vi "Preview Test Node.vi"(8 "error in (no error)":errorcluster, 11 "Test Node Model in":refnum<class "Test Node Model.lvclass">) -> (0 "error out":errorcluster, 3 "Test Node Model out":refnum<class "Test Node Model.lvclass">)   [LabVIEW 2013, in "Test Node Model.lvlib" / "Test Node Model.lvclass"]
uses:
  Test Node Model.lvclass
  Test Node Model.lvclass/Test Node Model.ctl
  <vilib>/xml/Load XML File.vi
  <vilib>/xml/Close Reference(Node).vi
  <vilib>/xml/NI_XML.lvlib
  Common/File IO/File IO.lvlib
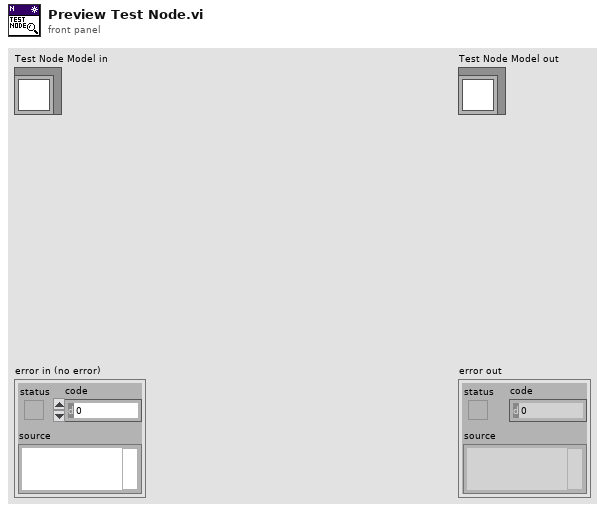
[diagram p1: front panel]
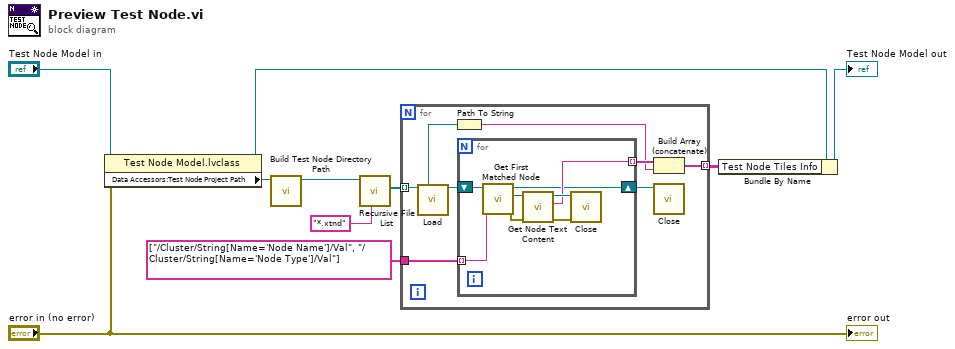
[diagram p0: block diagram]
diagram:
  n1 = property class="Test Node Model.lvclass"(reference="Test Node Model in", error in="error in (no error)") -> (reference out=w8:refnum<class "Test Node Model.lvclass">, "Data Accessors:Test Node Project Path"=w5:path)  [unwired: 1 out]
  n2 = call "Build Test Node Directory Path.vi"("Project Path"=w5) -> ("Test Node Directory Path"=w1:path)  [unwired: 10 in]
  n3 = call <vilib>:"Recursive File List.vi"("pattern"="*.xtnd", "Folder Path"=w1) -> ("All Files in Dir"=w2:path[])  [unwired: 5 in, 4 out]
  n4 = for {
    tunnel: w2 -> [w14] mode=indexing
    tunnel: string[] ["/Cluster/String[Name='Node Name']/Val", "/Cluster/String[Name='Node Type']/Val"] -> [w16]
    tunnel: [w11] -> w3 mode=indexing
    n5 = call-poly <vilib>:"Load.vi"("path to XML document"=w14) -> ("DOM document out"=w17:refnum<k20>)  [unwired: 12 in, 2 out]
    n6 = Path To String(path=w14) -> (string=w13:string)
    n7 = for {
      shift-right: [w18] -> w12
      shift-left: w17 -> [w25]
      tunnel: w16 -> [w24] mode=indexing
      tunnel: [w21] -> w15 mode=indexing
      n8 = call <vilib>:"Get First Matched Node.vi"("XPath expression"=w24, "node in"=w25) -> ("error out"=w19:errorcluster, "node result"=w23:refnum<k20>, "node out"=w18:refnum<k20>)  [unwired: 7 in]
      n9 = call <vilib>:"Get Node Text Content.vi"("error in (no error)"=w19, "node in"=w23) -> ("error out"=w20:errorcluster, "node text"=w21:string, "node out"=w22:refnum<k20>)  [unwired: 7 in]
      n10 = call-poly <vilib>:"Close.vi"("error in (no error)"=w20, "node"=w22) -> ()  [unwired: 7 in, 1 out]
    }
    n11 = Build Array (concatenate)(w15, w13) -> (w11:string[])
    n12 = call-poly <vilib>:"Close.vi"("node"=w12) -> ()  [unwired: 8 in, 1 out]
  }
  n13 = Bundle By Name(cluster=w8, "Test Node Tiles Info"=w3) -> (→"Test Node Model out":refnum<class "Test Node Model.lvclass">)
  "error out" <- "error in (no error)"
